vi "Module Loop.vi"(8 "error in (no error)":errorcluster, 11 "ToggleTestModule in":refnum<class "ToggleTestModule.lvclass">) -> (0 "error out":errorcluster, 3 "ToggleTestModule out":refnum<class "ToggleTestModule.lvclass">)   [LabVIEW 2020, in "VolatusScratch.lvlib" / "ToggleTestModule.lvclass"]
uses:
  ToggleTestModule.lvclass
  C:/dev/lv20CE/relink/lv-volatus/Volatus/Module/Module.lvclass
  Volatus/Module/Module.lvclass/Module.ctl
  Volatus/Module/Module.lvclass
  lv-vecto/Vecto/proto/Empty/Class/Msg.lvclass
  C:/dev/lv20CE/relink/lv-protoc/LV-Proto/Message/Message.lvclass
  Volatus/VolatusAPI/VolatusAPI.lvclass/VolatusAPI.ctl
  messages/TwoDoubles/Class/Msg.lvclass/Msg.ctl
  Volatus/MessageQ/MessageQ.lvclass/MessageQ.ctl
  messages/TwoDoubles/Class/Msg.lvclass
  lv-vecto/Vecto/TCPMessageService/Send Message.vi
  <vilib>/Utility/error.llb/Error Cluster From Error Code.vi
  lv-protoc/LV-Proto/Message/Message.lvclass
  ToggleTestModule.lvclass/ToggleTestModule.ctl
  Volatus/MessageQ/MessageQ.lvclass
  Volatus/VolatusAPI/VolatusAPI.lvclass
  Volatus/Volatus.lvlib
  messages/Double/Double.lvlib
panel:
  out "Timeout":bool
  in  "Compute":bool
  out "c":dbl
  in  "b":dbl
  in  "a":dbl
  in  "Generic Toggle":bool
  # "^2"
  # "^2"
  # "^2"
  # "+"
  # "="
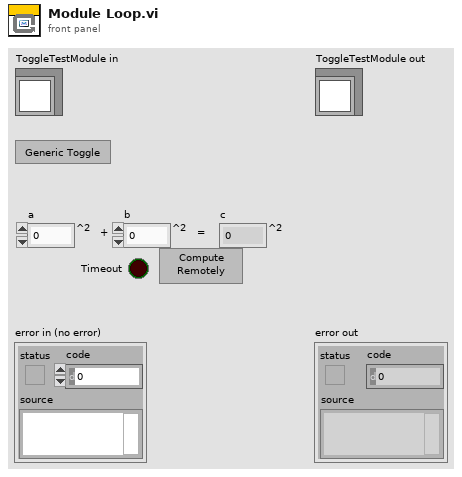
[diagram p1: front panel]
types:
  T1 = enum32{"Invalid", "Standard", "Closed", "Hidden", "Minimized", "Maximized"}
  T2 = enum8{"Enabled", "Disabled", "Disabled and Grayed Out"}
  T3 = typedef "TcpPayload.lvlib/Data.ctl" = cluster{"target_node":u32, "source_id":u32, "sequence":u32, "timestamp":u64, "type":string, "task_id":string, "payload":u8[]}
  T4 = typedef "Double.lvlib/Data.ctl" = cluster{"a":dbl}
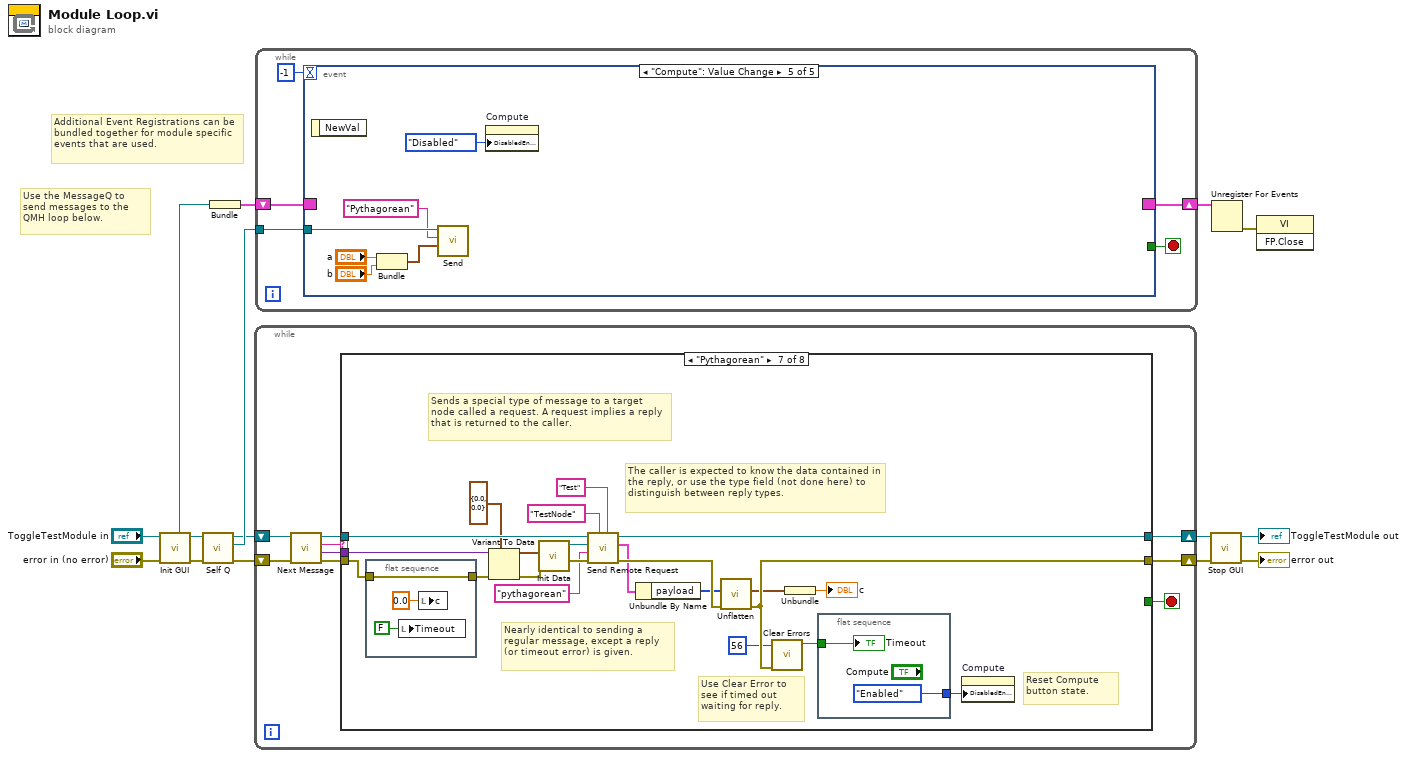
[diagram p0: block diagram]
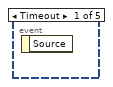
[diagram p2: hidden frame]
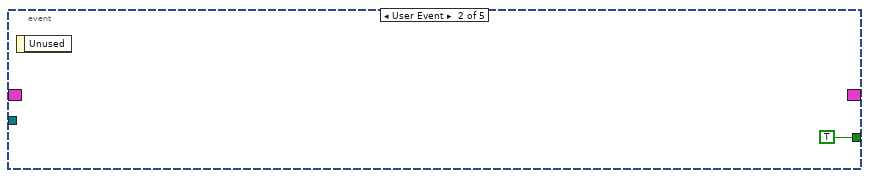
[diagram p3: hidden frame]
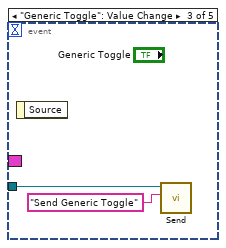
[diagram p4: hidden frame]
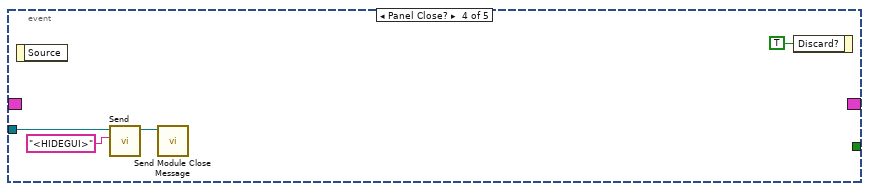
[diagram p5: hidden frame]
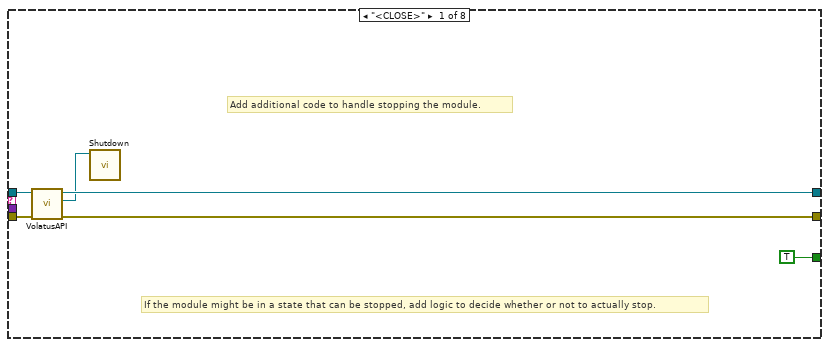
[diagram p6: hidden frame]
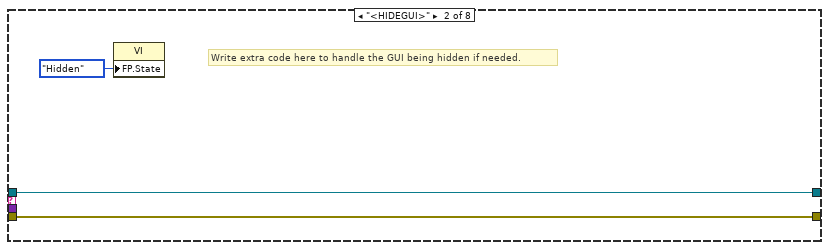
[diagram p7: hidden frame]
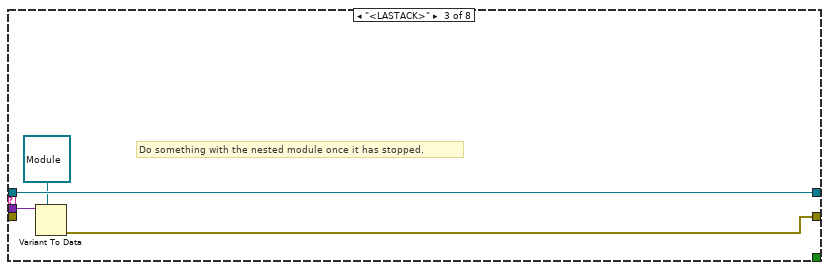
[diagram p8: hidden frame]
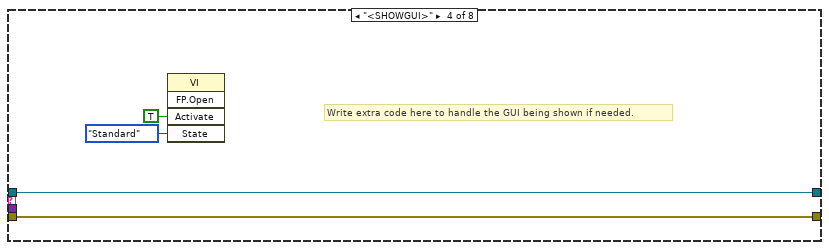
[diagram p9: hidden frame]
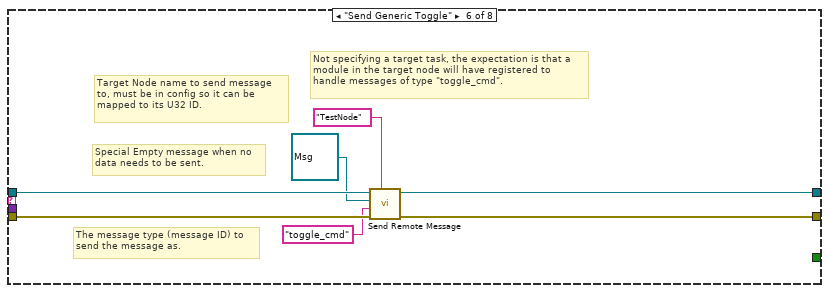
[diagram p11: hidden frame]
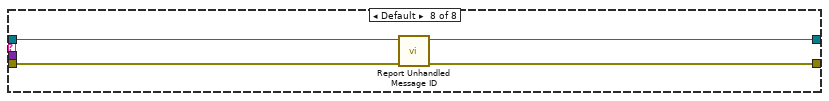
[diagram p12: hidden frame]
diagram:
  # "Additional Event Registrations can be bundled together for module specific events that are used."
  # "Use the MessageQ to send messages to the QMH loop below."
  n1 = call "Init GUI.vi"("Module in"="ToggleTestModule in") -> ("Module out"=w7:refnum<class "ToggleTestModule.lvclass">, "Event Reg"=w12:refnum<event-registration>)  [unwired: 9 in]
  n2 = call "Self Q.vi"("Module in"=w7) -> ("Self Q"=w6:refnum<class "MessageQ.lvclass">, "Module out"=w5:refnum<class "ToggleTestModule.lvclass">)  [unwired: 9 in]
  n3 = Bundle("Event Reg"=w12) -> (w8:cluster{"Event Reg":refnum<event-registration>})  [unwired: 1 in]
  n4 = while {
    shift-right: [w17] -> w10
    shift-left: w5 -> [w22]
    shift-right: [w16] -> w11
    shift-left: "error in (no error)" -> [w21]
    stop <- w15 stop-if-true
    n5 = call "Next Message.vi"("error in (no error)"=w21, "Module in"=w22) -> ("error out"=w20:errorcluster, "Data"=w14:variant, "ID"=w19:string, "Module out"=w18:refnum<class "ToggleTestModule.lvclass">)  [unwired: 6 in]
    n6 = case shown="\"Pythagorean\"" w19 {
      tunnel: w20 -> [w25 w29 _ w37 w39 w47 w50 w77]
      tunnel: w18 -> [w26 w30 w34 w38 w40 w45 w65 w75]
      tunnel: [w24 w30 w34 w38 w40 w44 w61 w74] -> w17
      tunnel: [w25 w29 w31 w37 w39 w46 w68 w76] -> w16
      tunnel: [TRUE _ _ _ _ _ _ _] -> w15
      tunnel: w14 -> [_ _ w33 _ _ _ w64 _]
      frame "<CLOSE>" {
        # "If the module might be in a state that can be stopped, add logic to decide whether or not to actually stop."
        # "Add additional code to handle stopping the module."
        n7 = call "VolatusAPI.vi"("Module in"=w26) -> ("VolatusAPI"=w23:refnum<class "VolatusAPI.lvclass">, "Module out"=w24:refnum<class "ToggleTestModule.lvclass">)  [unwired: 9 in]
        n8 = call "Shutdown.vi"("VolatusAPI in"=w23) -> ()  [unwired: 9 in, 2 out]
      }
      frame "<HIDEGUI>" {
        # "Write extra code here to handle the GUI being hidden if needed."
        n9 = property class="VI"("FP.State"=T1."Hidden" ("Front Panel Window:State")) -> ()  [unwired: 2 in, 2 out]
      }
      frame "<LASTACK>" {
        # "Do something with the nested module once it has stopped."
        n10 = Variant To Data(type=refnum<class "Module.lvclass"> refnum ("Volatus:Module"), Variant=w33) -> (error out=w31:errorcluster)  [unwired: 1 in, 1 out]
      }
      frame "<SHOWGUI>" {
        # "Write extra code here to handle the GUI being shown if needed."
        n11 = invoke class="VI" method="FP.Open"("Activate"=TRUE ("Activate?"), "State"=T1."Standard") -> ()  [unwired: 3 in, 5 out]
      }
      frame "<TIMEOUT>" {
        # "No message for this module was received in time"
      }
      frame "Send Generic Toggle" {
        # "Not specifying a target task, the expectation is that a module in the target node will have registered to handle messages of type \"toggle_cmd\"."
        # "The message type (message ID) to send the message as."
        # "Target Node name to send message to, must be in config so it can be mapped to its U32 ID."
        # "Special Empty message when no data needs to be sent."
        n12 = call "Send Remote Message.vi"("Target Node"="TestNode", "error in (no error)"=w47, "Message Type"="toggle_cmd", "Message"=refnum<class "Msg.lvclass"> refnum ("Empty.lvlib:Msg.lvclass"), "Module in"=w45) -> ("error out"=w46:errorcluster, "Module out"=w44:refnum<class "ToggleTestModule.lvclass">)  [unwired: 5 in]
      }
      frame "Pythagorean" {
        # "Reset Compute button state."
        # "Use Clear Error to see if timed out waiting for reply."
        # "Nearly identical to sending a regular message, except a reply (or timeout error) is given."
        # "The caller is expected to know the data contained in the reply, or use the type field (not done here) to distinguish between reply types."
        # "Sends a special type of message to a target node called a request. A request implies a reply that is returned to the caller."
        n13 = flat-sequence {
          tunnel: [w73] -> w51
          tunnel: w50 -> [w73]
          frame #0 {
            n14 = local write "Timeout"(FALSE ("Timeout")) -> ()
            n15 = local write "c"(0.0 ("c")) -> ()
          }
        }
        n16 = Variant To Data(error in=w51, type=cluster{"a":dbl, "b":dbl} {"a"=0.0, "b"=0.0} ("cluster"), Variant=w64) -> (data=w62:cluster{"a":dbl, "b":dbl}, error out=w66:errorcluster)
        n17 = call "Init Data.vi"("Data"=w62) -> ("Msg out"=w59:refnum<class "Msg.lvclass">)  [unwired: 10 in]
        n18 = call "Send Remote Request.vi"("Target Task (None)"="Test" ("Target Node"), "Target Node"="TestNode", "error in (no error)"=w66, "Message Type"="pythagorean", "Message"=w59, "Module in"=w65) -> ("error out"=w67:errorcluster, "Reply"=w57:T3, "Module out"=w61:refnum<class "ToggleTestModule.lvclass">)  [unwired: 3 in]
        n19 = Unbundle By Name(w57) -> ("payload"=w56:u8[])
        n20 = call "Unflatten.vi"("error in"=w67, "Buffer"=w56) -> ("error out"=w68:errorcluster, "Data"=w55:T4)  [unwired: 8 in]
        n21 = call <vilib>:"Clear Errors.vi"("error in (no error)"=w68, "specific error code to clear (0: all)"=56) -> ("specific error cleared?"=w52:bool)  [unwired: 4 in, 1 out]
        n22 = Unbundle(w55) -> ("a"=→"c":dbl)
        n23 = flat-sequence {
          tunnel: w52 -> [w70]
          tunnel: [T2."Enabled" ("Disabled")] -> w49
          frame #0 {
            "Timeout" <- w70
          }
        }
        n24 = property on="Compute" class="Bool"("DisabledEnum"=w49) -> ()  [unwired: 2 in, 2 out]
      }
      frame Default {
        n25 = call "Report Unhandled Message ID.vi"("error in (no error)"=w77, "Module in"=w75) -> ("error out"=w76:errorcluster, "Module out"=w74:refnum<class "ToggleTestModule.lvclass">)  [unwired: 8 in]
      }
    }
  }
  n26 = while {
    tunnel: w6 -> [w82]
    shift-right: [w80] -> w9
    shift-left: w8 -> [w81]
    stop <- w79 stop-if-true
    n27 = event shown="[4] \"Compute\": Value Change" {
      selector: w81 -> [_ _ _ _ _]
      dyn-events: [_ _ _ _ _] -> w80
      timeout: -1 -> [_ _ _ _ _]
      tunnel: w82 -> [_ _ w85 w88 w93]
      tunnel: [_ TRUE _ _ _] -> w79
      event Timeout {
        n28 = event-data() -> ()  [unwired: 1 in, 1 out]
      }
      event User Event {
        n29 = event-data() -> ()  [unwired: 1 in, 1 out]
      }
      event "Generic Toggle": Value Change {
        n30 = event-data() -> ()  [unwired: 1 in, 1 out]
        n31 = call "Send.vi"("ID"="Send Generic Toggle", "MessageQ in"=w85) -> ()  [unwired: 8 in, 2 out]
      }
      event Panel Close? {
        n32 = event-data() -> ()  [unwired: 1 in, 1 out]
        n33 = call "Send.vi"("ID"="<HIDEGUI>", "MessageQ in"=w88) -> ("MessageQ out"=w86:refnum<class "MessageQ.lvclass">)  [unwired: 8 in, 1 out]
        n34 = call "Send Module Close Message.vi"("MessageQ"=w86) -> ()  [unwired: 10 in, 1 out]
        n35 = event-data("Discard?"=TRUE) -> ()  [unwired: 1 in, 1 out]
      }
      event "Compute": Value Change {
        n36 = event-data() -> ()  [unwired: 1 in, 1 out]
        n37 = Bundle("a"="a", "b"="b") -> (w92:cluster{"a":dbl, "b":dbl})  [unwired: 1 in]
        n38 = call "Send.vi"("Data"=w92, "ID"="Pythagorean", "MessageQ in"=w93) -> ()  [unwired: 7 in, 2 out]
        n39 = property on="Compute" class="Bool"("DisabledEnum"=T2."Disabled" ("Disabled")) -> ()  [unwired: 2 in, 2 out]
      }
    }
  }
  n40 = call "Stop GUI.vi"("error in (no error)"=w11, "Module in"=w10) -> ("error out"=→"error out":errorcluster, "Module out"=→"ToggleTestModule out":refnum<class "ToggleTestModule.lvclass">)  [unwired: 8 in]
  n41 = Unregister For Events(event registration refnum=w9) -> (error out=w13:errorcluster)  [unwired: 1 in]
  n42 = invoke class="VI" method="FP.Close"(error in=w13) -> ()  [unwired: 2 in, 3 out]
